vi "TEST_bench_FXP_Matrix-Vector_mult_loop_32bit.vi"(6 "NS":u8=9, 8 "Az_col":fxp<+/-,32,5>[](array[numeric])=[0.0, 0.0, 0.0, 0.0, 0.0, 0.0, 0.0, 0.0, 0.0, 0.0, 0.0, 0.0, 0.0, 0.0, 0.0, 0.0, 0.0, 0.0, 0.0, 0.0, 0.0, 0.0, 0.0, 0.0, 0.0, 0.0, 0.0, 0.0, 0.0, 0.0, 0.0, 0.0, 0.0, 0.0, 0.0, 0.0, 0.0, 0.0, 0.0, 0.0, 0.0, 0.0, 0.0, 0.0, 0.0, 0.0, 0.0, 0.0, 0.0, 0.0], 11 "x_k":fxp<+/-,32,5>[](array[numeric])=[0.0, 0.0, 0.0, 0.0, 0.0, 0.0, 0.0, 0.0, 0.0, 0.0, 0.0, 0.0, 0.0, 0.0, 0.0, 0.0, 0.0, 0.0, 0.0, 0.0, 0.0, 0.0, 0.0, 0.0, 0.0, 0.0, 0.0, 0.0, 0.0, 0.0, 0.0, 0.0, 0.0, 0.0, 0.0, 0.0, 0.0, 0.0, 0.0, 0.0, 0.0, 0.0, 0.0, 0.0, 0.0, 0.0, 0.0, 0.0, 0.0, 0.0]) -> (0 "xk_0_1":T1, 3 "Ax (xk_1_0)":T1)   [LabVIEW 2017]
uses:
  fpga_subVIs_ssxy/fixed-point-ss/typeDefs/x_vec_type.ctl
  fpga_subVIs_ssxy/fixed-point-ss/typeDefs/x_vec_bram.ctl
  fpga_subVIs_ssxy/fixed-point-ss/typeDefs/A_as_vec_bram.ctl
  <vilib>/rvi/DataTransferAndStorage/Container/Common/niFpgaContainerExecOnDevCompGetState.vi
  <vilib>/rvi/Emulation/niFpgaEmulationIsFPGAContextNoSignature.vi
  <vilib>/rvi/DataTransferAndStorage/Container/Common/niFpgaContainerGetUniqueNameForEmu.vi
  <vilib>/rvi/Emulation/niFpgaProcessEmulError.vi
  <vilib>/rvi/Emulation/niFpgaSctlEmulationGetInTimedLoop.vi
  <vilib>/rvi/errors/nirviReportUnexpectedCaseInternalError (U32).vi
  <vilib>/rvi/Memory/Memory_Emulation/niFpgaMemoryEmulationCacheClearOnFirstRun.vi
  <vilib>/rvi/Memory/Memory_Emulation/nirvimemoryEmulationManagerCache_MakeExclusive.vi
  <vilib>/rvi/Memory/Memory_Emulation/niFpgaMemoryEmulationValidateCache.vi
  <vilib>/rvi/Memory/Memory_Emulation/nirvimemoryEmulationManagerCache_InsertValue.vi
  <vilib>/Utility/error.llb/Clear Errors.vi
  <vilib>/rvi/Memory/Memory_Emulation/nirvimemoryEmulationManagerCache_ReleaseExclusive.vi
  <vilib>/rvi/Memory/Memory_Emulation/nirvimemoryEmulationManagerCache_GetValue.vi
  <vilib>/rvi/Memory/Memory_Emulation/nirvimemoryEmulationManagerCache_SetValue.vi
  <vilib>/rvi/Emulation/niFpgaSctlEmulationResourceMgr.vi
  <vilib>/rvi/DataTransferAndStorage/Container/XNode/niFpgaContainer.xnode
  <vilib>/rvi/Memory/Memory_Emulation/niFpgaMemoryEmulationRefIn.vi
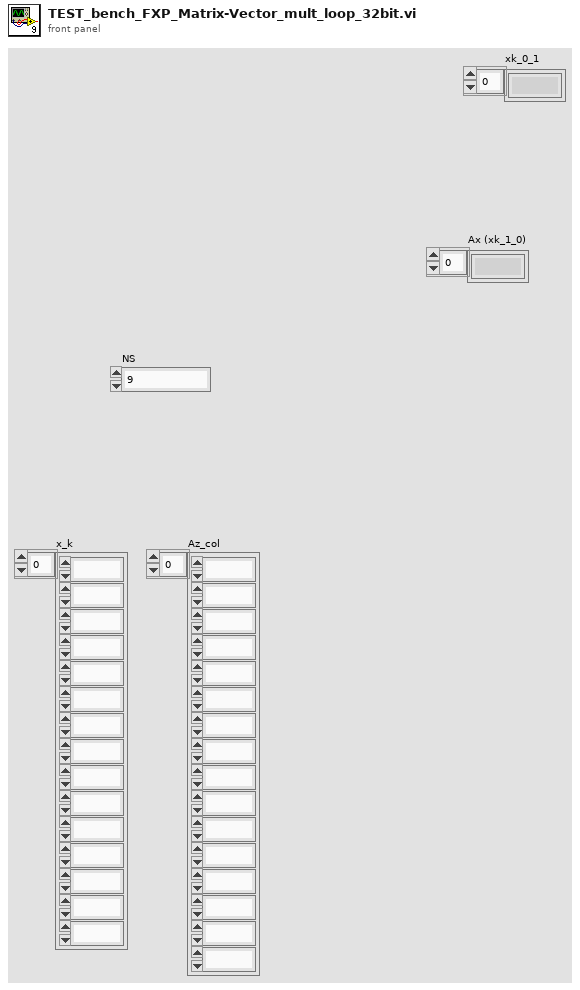
[diagram p1: front panel]
types:
  T1 = typedef "x_vec_type.ctl" = fxp<+/-,32,6>[]
  T2 = typedef "x_vec_bram.ctl" = refnum<k21>
  T3 = typedef "A_as_vec_bram.ctl" = refnum<k21>
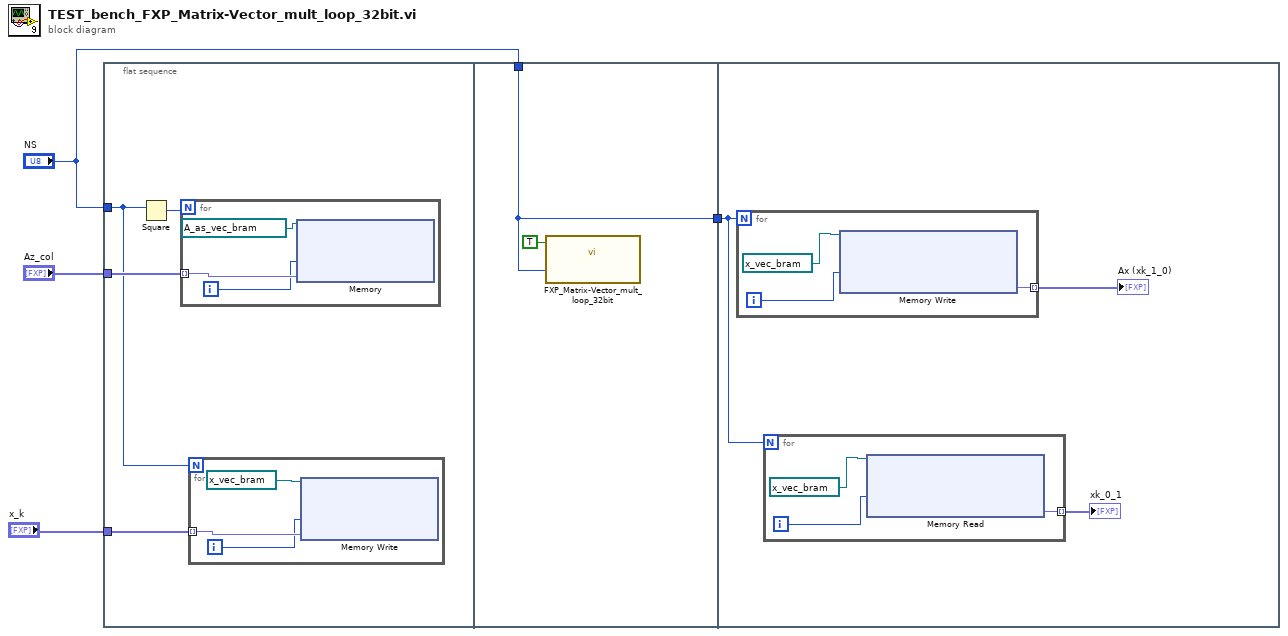
[diagram p0: block diagram]
diagram:
  n1 = flat-sequence {
    tunnel: "NS" -> [w5]
    tunnel: "Az_col" -> [w8]
    tunnel: "x_k" -> [w7]
    tunnel: "NS" -> [w16]
    tunnel: [w16] -> w1
    tunnel: w1 -> [w18]
    frame #0 {
      n2 = Square(x=w5) -> (x^2=w6:u8)
      n3 = for {
        N: w6 -> [_]
        tunnel: w8 -> [w14] mode=indexing
        i -> [w13]
        n4 = xnode "Memory"("Address"=w13, "Data"=w14, "Memory In"=T3 "AasCol _FXP") -> ()  [unwired: 1 out]
      }
      n5 = for {
        N: w5 -> [_]
        tunnel: w7 -> [w11] mode=indexing
        i -> [w10]
        n6 = xnode "Memory Write"("Address"=w10, "Data"=w11, "Memory In"=T2 "xk_0_1" ("Memory")) -> ()  [unwired: 1 out]
      }
    }
    frame #1 {
      n7 = call "FXP_Matrix-Vector_mult_loop_32bit.vi"("Ns_1"=w16, "inputValid"=TRUE) -> ()  [unwired: 9 in, 1 out]
    }
    frame #2 {
      n8 = for {
        N: w18 -> [_]
        tunnel: [w24] -> w19 mode=indexing
        i -> [w25]
        n9 = xnode "Memory Write"("Address"=w25, "Memory In"=T2 "xk_1_0" ("Memory")) -> ("Data"=w24:fxp<+/-,32,6>)  [unwired: 1 out]
      }
      "Ax (xk_1_0)" <- w19
      n10 = for {
        N: w18 -> [_]
        tunnel: [w21] -> w17 mode=indexing
        i -> [w22]
        n11 = xnode "Memory Read"("Address"=w22, "Memory In"=T2 "xk_0_1" ("Memory")) -> ("Data"=w21:fxp<+/-,32,6>)  [unwired: 1 out]
      }
      "xk_0_1" <- w17
    }
  }
